vi "WriteFrontPanelToFrameworkIni.vi"(8 "ErrorArray In":errorcluster[](array[cluster]), 10 "clFrontPanelControlRefs In":T1) -> (0 "ErrorArray Out":errorcluster[](array[cluster]), 2 "clFrontPanelControlRefs Out":T1)   [LabVIEW 2014]
uses:
  <userlib>/NIST/NISTErrorLib/NISTErrorLib.lvlib
  Config.lvclass
  <vilib>/Utility/config.llb/NI_LVConfig.lvlib
  <vilib>/Utility/config.llb/Write Key (String).vi
  <vilib>/Utility/config.llb/Write Key (Path).vi
  FrontPanel/TypeDefs/clEventConfig.ctl
  Framework.lvlib
  FrontPanel/TypeDefs/clFrontPanelControlRefs.ctl
  Modules/PmuImpairPlugins/PmuImpairPluginBase_class/TypeDefs/clImpairConfig.ctl
  Modules/PmuImpairPlugins/PmuImpairPluginBase_class/PmuImpairPluginBase.lvclass
panel:
  # "When you add a control \non the front panel, add a\nreference for it in this\ntype def.  This cluster\nwill hold all of the refer-\nences to the front panel\ncontrols in order to pass\nthese control references \nto subvis."
  # "When you add a control \non the front panel, add a\nreference for it in this\ntype def.  This cluster\nwill hold all of the refer-\nences to the front panel\ncontrols in order to pass\nthese control references \nto subvis."
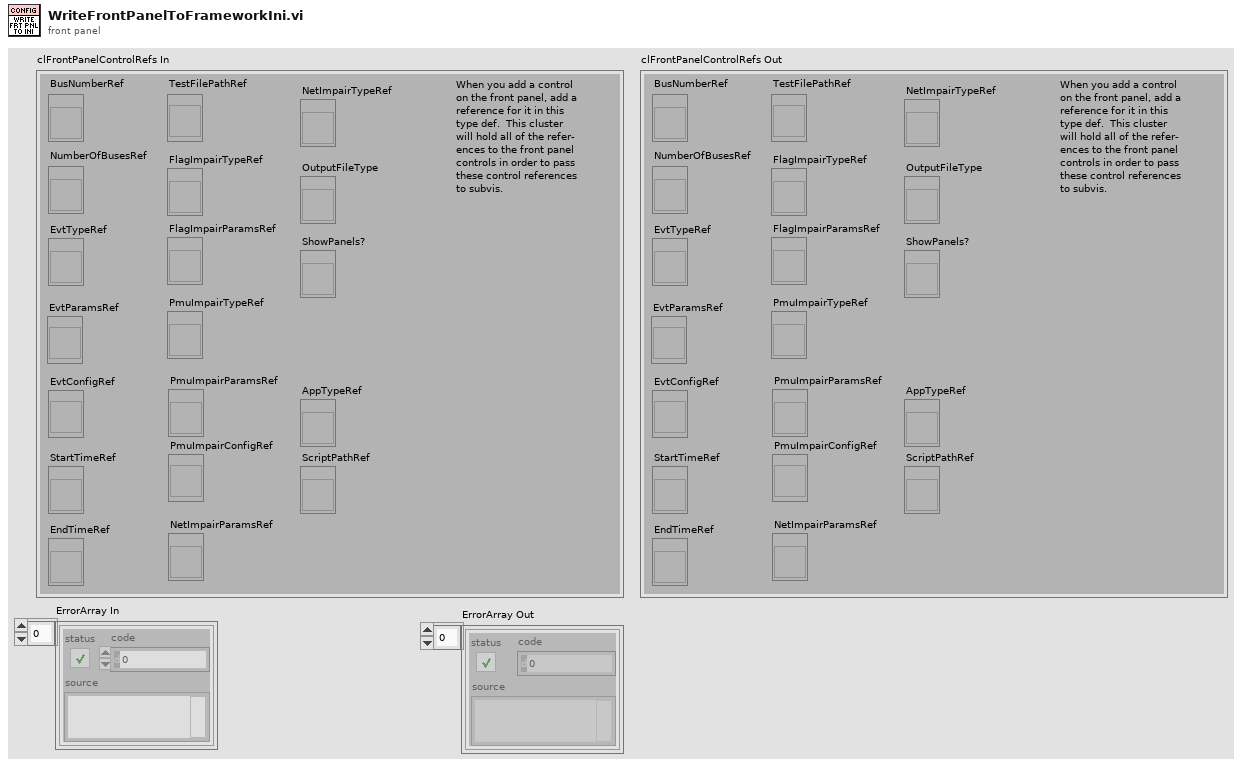
[diagram p1: front panel]
types:
  T1 = typedef "Framework.lvlib/clFrontPanelControlRefs.ctl" = cluster{"TestFilePathRef":refnum<vi>, "BusNumberRef":refnum<vi>, "NumberOfBusesRef":refnum<vi>, "EvtTypeRef":refnum<vi>, "EvtParamsRef":refnum<vi>, "EvtConfigRef":refnum<vi>, "StartTimeRef":refnum<vi>, "EndTimeRef":refnum<vi>, "PmuImpairTypeRef":refnum<vi>, "PmuImpairParamsRef":refnum<vi>, "NetImpairParamsRef":refnum<vi>, "FlagImpairTypeRef":refnum<vi>, "FlagImpairParamsRef":refnum<vi>, "NetImpairTypeRef":refnum<vi>, "OutputFileType":refnum<vi>, "PmuImpairConfigRef":refnum<vi>, "AppTypeRef":refnum<vi>, "ScriptPathRef":refnum<vi>, "ShowPanels?":refnum<vi>}
  T2 = typedef "PmuImpairPlugins.lvlib/PmuImpairPluginBase.lvclass/clImpairConfig.ctl" = cluster{"FilterType":string, "bPosSeq":bool}
  T3 = typedef "Framework.lvlib/clEventConfig.ctl" = cluster{"UTC Time 0":timestamp, "Nominal Frequency":u16, "Reporting Rate":u16, "Fsamp":u32, "PosSeq":bool}
  T4 = typedef "LVStringsAndValuesArrayTypeDef_U16.ctl" = cluster{"String":string, "Value":u16}[]
  T5 = typedef "NI_LVConfig.lvlib/Config Data RefNum.ctl" = refnum<k1>
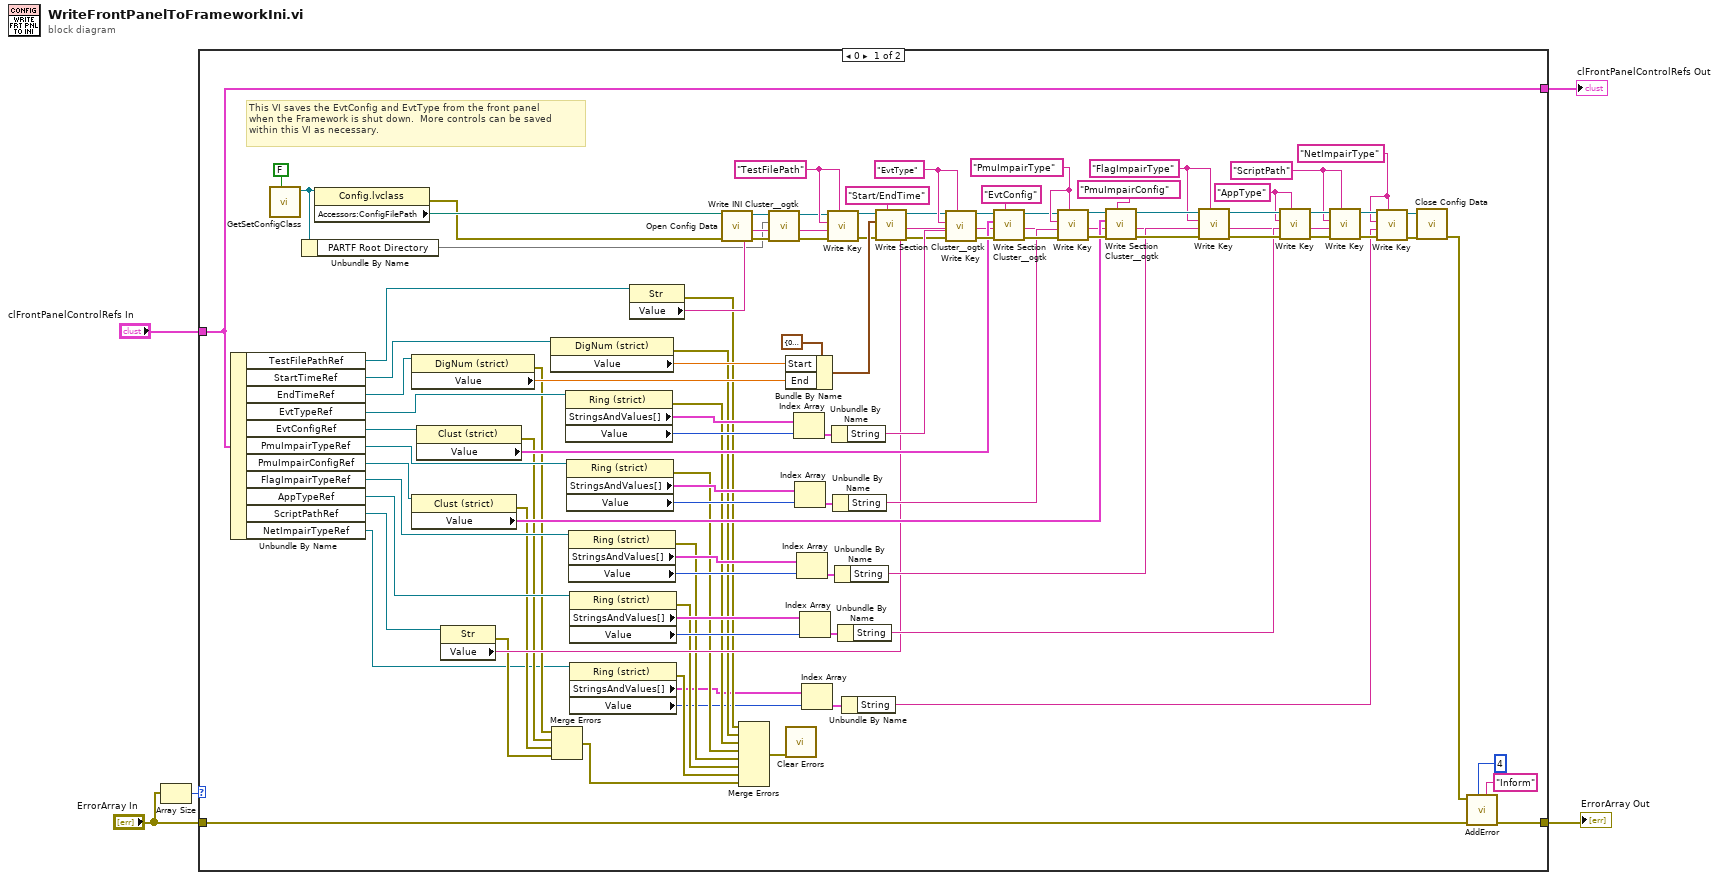
[diagram p0: block diagram]
diagram:
  n1 = Array Size(array="ErrorArray In") -> (size(s)=w3:i32)
  n2 = case shown="0" w3 {
    tunnel: [w100 w104] -> w5
    tunnel: "ErrorArray In" -> [w99 w104]
    tunnel: "clFrontPanelControlRefs In" -> [w91 w103]
    tunnel: [w91 w103] -> w1
    frame 0 {
      w7 = "NetImpairType" ("key")
      w36 = "ScriptPath" ("key")
      w41 = "AppType" ("section")
      w54 = "FlagImpairType" ("key")
      w57 = "TestFilePath" ("key")
      w79 = "PmuImpairType" ("key")
      w94 = "EvtType" ("key")
      # "This VI saves the EvtConfig and EvtType from the front panel\nwhen the Framework is shut down.  More controls can be saved\nwithin this VI as necessary."
      n3 = Unbundle By Name(w91) -> ("TestFilePathRef"=w60:refnum<vi>, "StartTimeRef"=w69:refnum<vi>, "EndTimeRef"=w68:refnum<vi>, "EvtTypeRef"=w95:refnum<vi>, "EvtConfigRef"=w86:refnum<vi>, "PmuImpairTypeRef"=w74:refnum<vi>, "PmuImpairConfigRef"=w73:refnum<vi>, "FlagImpairTypeRef"=w51:refnum<vi>, "AppTypeRef"=w45:refnum<vi>, "ScriptPathRef"=w39:refnum<vi>, "NetImpairTypeRef"=w17:refnum<vi>)
      n4 = call "GetSetConfigClass.vi"("Set (f)"=FALSE) -> ("Ref out"=w19:refnum<class "Config.lvclass">)  [unwired: 10 in]
      n5 = Unbundle By Name(w19) -> ("PARTF Root Directory"=w18)
      n6 = property class="Config.lvclass"(reference=w19) -> (error out=w96:errorcluster, "Accessors:ConfigFilePath"=w97:path)  [unwired: 1 in, 1 out]
      n7 = property class="DigNum (strict)"(reference=w68) -> (error out=w34:errorcluster, "Value"=w63:dbl)  [unwired: 1 in, 1 out]
      n8 = property class="Clust (strict)"(reference=w73) -> (error out=w32:errorcluster, "Value"=w71:T2)  [unwired: 1 in, 1 out]
      n9 = property class="Clust (strict)"(reference=w86) -> (error out=w33:errorcluster, "Value"=w83:T3)  [unwired: 1 in, 1 out]
      n10 = property class="Str"(reference=w39) -> (error out=w31:errorcluster, "Value"=w35:string)  [unwired: 1 in, 1 out]
      n11 = property class="DigNum (strict)"(reference=w69) -> (error out=w30:errorcluster, "Value"=w64:dbl)  [unwired: 1 in, 1 out]
      n12 = Merge Errors(w34, w33, w32, w31) -> (w15:errorcluster)
      n13 = property class="Ring (strict)"(reference=w95) -> (error out=w29:errorcluster, "StringsAndValues[]"=w89:T4, "Value"=w90:u16)  [unwired: 1 in, 1 out]
      n14 = property class="Ring (strict)"(reference=w74) -> (error out=w28:errorcluster, "StringsAndValues[]"=w76:T4, "Value"=w75:u16)  [unwired: 1 in, 1 out]
      n15 = property class="Ring (strict)"(reference=w51) -> (error out=w27:errorcluster, "StringsAndValues[]"=w53:T4, "Value"=w52:u16)  [unwired: 1 in, 1 out]
      n16 = property class="Ring (strict)"(reference=w45) -> (error out=w26:errorcluster, "StringsAndValues[]"=w47:T4, "Value"=w46:u16)  [unwired: 1 in, 1 out]
      n17 = property class="Ring (strict)"(reference=w17) -> (error out=w16:errorcluster, "StringsAndValues[]"=w14:T4, "Value"=w13:u16)  [unwired: 1 in, 1 out]
      n18 = property class="Str"(reference=w60) -> (error out=w24:errorcluster, "Value"=w48:string)  [unwired: 1 in, 1 out]
      n19 = call <vilib>:"Open Config Data.vi"("error in (no error)"=w96, "configuration file path"=w97) -> ("error out"=w23:errorcluster, "refnum"=w22:T5)  [unwired: 7 in, 1 out]
      n20 = Merge Errors(w24, w30, w29, w28, w27, w26, w16, w15) -> (w25:errorcluster)
      n21 = call <userlib>:"Write INI Cluster__ogtk.vi"("error in (no error)"=w23, "INI Fomatted Cluster"=w18, "refnum"=w22) -> ("error out"=w20:errorcluster, "dup refnum"=w21:T5)  [unwired: 7 in]
      n22 = Bundle By Name(cluster=cluster{"Start":dbl, "End":dbl} {"Start"=0.0, "End"=0.0} ("Start/EndTime"), "Start"=w64, "End"=w63) -> (w62:cluster{"Start":dbl, "End":dbl})
      n23 = call <vilib>:"Clear Errors.vi"("error in (no error)"=w25) -> ()  [unwired: 5 in, 2 out]
      n24 = Index Array(array=w89, index=w90) -> (element=w88:cluster{"String":string, "Value":u16})
      n25 = Index Array(array=w76, index=w75) -> (element=w77:cluster{"String":string, "Value":u16})
      n26 = Index Array(array=w53, index=w52) -> (element=w50:cluster{"String":string, "Value":u16})
      n27 = Index Array(array=w47, index=w46) -> (element=w44:cluster{"String":string, "Value":u16})
      n28 = Index Array(array=w14, index=w13) -> (element=w12:cluster{"String":string, "Value":u16})
      n29 = call-poly <vilib>:"Write Key.vi"("section"=w57, "error in (no error)"=w20, "value"=w48, "key"=w57, "refnum"=w21) -> ("error out"=w59:errorcluster, "refnum out"=w58:T5)  [unwired: 4 in, 1 out]
      n30 = Unbundle By Name(w88) -> ("String"=w87:string)
      n31 = Unbundle By Name(w77) -> ("String"=w72:string)
      n32 = Unbundle By Name(w50) -> ("String"=w49:string)
      n33 = Unbundle By Name(w44) -> ("String"=w40:string)
      n34 = Unbundle By Name(w12) -> ("String"=w6:string)
      n35 = call <userlib>:"Write Section Cluster__ogtk.vi"("section (optional)"="Start/EndTime", "error in (no error)"=w59, "Section Formatted Cluster"=w62, "refnum"=w58) -> ("error out"=w67:errorcluster, "dup refnum"=w65:T5)  [unwired: 6 in]
      n36 = call-poly <vilib>:"Write Key.vi"("section"=w94, "error in (no error)"=w67, "value"=w87, "key"=w94, "refnum"=w65) -> ("error out"=w84:errorcluster, "refnum out"=w85:T5)  [unwired: 4 in, 1 out]
      n37 = call <userlib>:"Write Section Cluster__ogtk.vi"("section (optional)"="EvtConfig", "error in (no error)"=w84, "Section Formatted Cluster"=w83, "refnum"=w85) -> ("error out"=w78:errorcluster, "dup refnum"=w70:T5)  [unwired: 6 in]
      n38 = call-poly <vilib>:"Write Key.vi"("section"=w79, "error in (no error)"=w78, "value"=w72, "key"=w79, "refnum"=w70) -> ("error out"=w82:errorcluster, "refnum out"=w81:T5)  [unwired: 4 in, 1 out]
      n39 = call <userlib>:"Write Section Cluster__ogtk.vi"("section (optional)"="PmuImpairConfig", "error in (no error)"=w82, "Section Formatted Cluster"=w71, "refnum"=w81) -> ("error out"=w55:errorcluster, "dup refnum"=w56:T5)  [unwired: 6 in]
      n40 = call-poly <vilib>:"Write Key.vi"("section"=w54, "error in (no error)"=w55, "value"=w49, "key"=w54, "refnum"=w56) -> ("error out"=w43:errorcluster, "refnum out"=w42:T5)  [unwired: 4 in, 1 out]
      n41 = call-poly <vilib>:"Write Key.vi"("section"=w41, "error in (no error)"=w43, "value"=w40, "key"=w41, "refnum"=w42) -> ("error out"=w38:errorcluster, "refnum out"=w37:T5)  [unwired: 4 in, 1 out]
      n42 = call-poly <vilib>:"Write Key.vi"("section"=w36, "error in (no error)"=w38, "value"=w35, "key"=w36, "refnum"=w37) -> ("error out"=w11:errorcluster, "refnum out"=w10:T5)  [unwired: 4 in, 1 out]
      n43 = call-poly <vilib>:"Write Key.vi"("section"=w7, "error in (no error)"=w11, "value"=w6, "key"=w7, "refnum"=w10) -> ("error out"=w9:errorcluster, "refnum out"=w8:T5)  [unwired: 4 in, 1 out]
      n44 = call <vilib>:"Close Config Data.vi"("error in (no error)"=w9, "refnum"=w8) -> ("error out"=w92:errorcluster)  [unwired: 8 in, 1 out]
      n45 = call <userlib>:"AddError.vi"("Severity"="Inform" ("String"), "Priority"=u8 4, "ErrorArray"=w99, "error in (no error)"=w92) -> ("ErrorArray"=w100:errorcluster[])  [unwired: 6 in, 1 out]
    }
    frame 1, Default {
    }
  }
  "clFrontPanelControlRefs Out" <- w1
  "ErrorArray Out" <- w5
